vi "readCommandExit.vi"(8 "error in (no error)":errorcluster, 10 "Parser":refnum<class "U8ArrayParserAutoIndexing.lvclass">, 11 "M1M3SAL in":refnum<class "M1M3SAL.lvclass">) -> (0 "error out":errorcluster, 2 "CommandExit":variant, 3 "M1M3SAL out":refnum<class "M1M3SAL.lvclass">)   [LabVIEW 2016, in "M1M3Communicator.lvlib" / "M1M3SAL.lvclass"]
uses:
  M1M3SAL.lvclass
  Common_RT_Utilities/U8ArrayParserAutoIndexing/U8ArrayParserAutoIndexing.lvclass
  Topics/CommandExit.ctl
  Topics/CommandId.ctl
  M1M3Communicator.lvlib
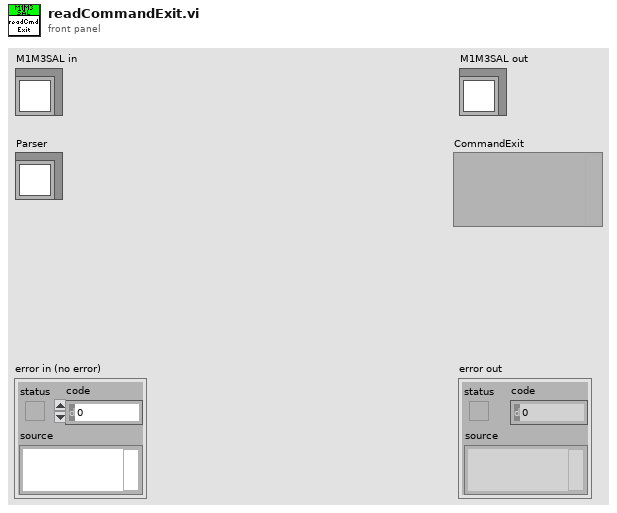
[diagram p1: front panel]
types:
  T1 = typedef "M1M3Communicator.lvlib/CommandExit.ctl" = cluster{"commandId":T2, "exitIsTrue":bool}
  T2 = typedef "M1M3Communicator.lvlib/CommandId.ctl" = i32
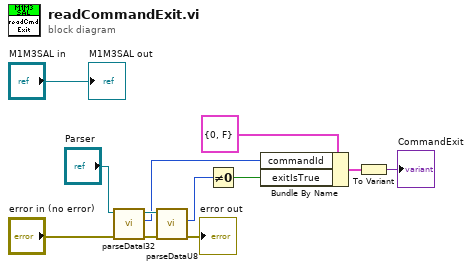
[diagram p0: block diagram]
diagram:
  n1 = call "parseDataI32.vi"("error in (no error)"="error in (no error)", "U8ArrayParserAutoIndexing in"="Parser") -> ("error out"=w3:errorcluster, "Data"=w1:i32, "U8ArrayParserAutoIndexing out"=w4:refnum<class "U8ArrayParserAutoIndexing.lvclass">)  [unwired: 7 in]
  n2 = call "parseDataU8.vi"("error in (no error)"=w3, "U8ArrayParserAutoIndexing in"=w4) -> ("error out"=→"error out":errorcluster, "Data"=w10:u8)  [unwired: 7 in, 1 out]
  n3 = Not Equal To 0?(x=w10) -> (x != 0?=w11:bool)
  n4 = Bundle By Name(cluster=T1 {"commandId"=0, "exitIsTrue"=FALSE} ("CommandExit"), "commandId"=w1, "exitIsTrue"=w11) -> (w7:T1)
  n5 = To Variant(anything=w7) -> (Variant=→"CommandExit":variant)
  "M1M3SAL out" <- "M1M3SAL in"
